vi "LSX Set Write Log Text FN.vi"(8 "error in (no error)":errorcluster, 9 "pcALogFN":string, 10 "bAWriteLogText":i32, 11 "lLSID":i32) -> (0 "error out":errorcluster, 1 "pcALogFN out":string, 3 "function return":i32)   [LabVIEW 2018, in "Tango.lvlib"]
doc: "TANGOAPI int TANGOCALL LSX_SetWriteLogTextFN (int lLSID, BOOL bAWriteLogText, char *pcALogFN);"
uses:
  <userlib>/Tango/Tango.lvlib
  <userlib>/Tango/Tango_DLL.dll
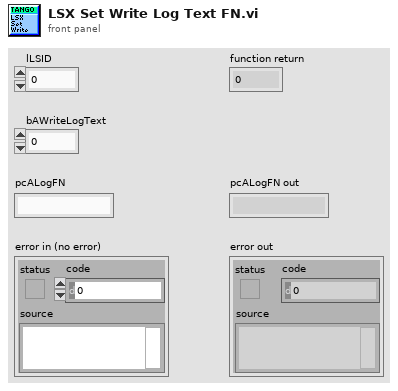
[diagram p1: front panel]
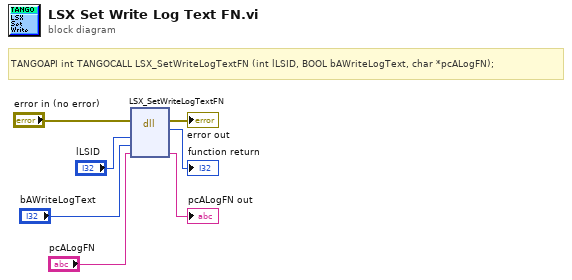
[diagram p0: block diagram]
diagram:
  # "TANGOAPI int TANGOCALL LSX_SetWriteLogTextFN (int lLSID, BOOL bAWriteLogText, char *pcALogFN);"
  n1 = dll-call lib="C:/Program Files (x86)/National Instruments/LabVIEW 2018/user.lib/Tango/Tango_DLL.*" fn="LSX_SetWriteLogTextFN"(error in="error in (no error)", "lLSID"="lLSID", "bAWriteLogText"="bAWriteLogText", "pcALogFN"="pcALogFN") -> (error out=→"error out":errorcluster, →"function return":i32, "pcALogFN"=→"pcALogFN out":string)  [unwired: 4 in, 1 out]
